vi "Configure Auth.vi"(8 "error in (no error)":errorcluster, 11 "SOL-Server in":refnum<class "SOL-Server.lvclass">) -> (0 "error out":errorcluster, 3 "SOL-Server out":refnum<class "SOL-Server.lvclass">)   [LabVIEW 2020, in "Summer of LabVIEW.lvlib" / "SOL-Server.lvclass"]
uses:
  SOL-Server.lvclass
  <vilib>/IlluminatedG/IG HTTP Server/HTTP Server/Optional Providers.ctl
  <vilib>/IlluminatedG/IG HTTP Server/HTTP Server/Password Encoder/Password Encoder.lvclass
  <vilib>/IlluminatedG/IG HTTP Server/HTTP Server/Authentication Provider/Authentication Provider.lvclass
  SOL-Server.lvclass/SOL-Server.ctl
  <vilib>/IlluminatedG/IG HTTP Server/HTTP Server/FormAuthentication/FormAuthentication.lvclass
  C:/Program Files (x86)/National Instruments/LabVIEW 2020/vi.lib/IlluminatedG/IG HTTP Server/HTTP Server/Authentication Provider/Authentication Provider.lvclass
  User DB/User DB.lvclass
  C:/Program Files (x86)/National Instruments/LabVIEW 2020/vi.lib/IlluminatedG/IG HTTP Server/HTTP Server/User Provider/User Provider.lvclass
  <vilib>/IlluminatedG/IG HTTP Server/HTTP Server/Server/Server.lvclass
  <vilib>/IlluminatedG/IG HTTP Server/HTTP Server/HTTP Server.lvlib
  SOL Auth/SOL Auth.lvclass
  C:/Program Files (x86)/National Instruments/LabVIEW 2020/vi.lib/IlluminatedG/IG HTTP Server/HTTP Server/Service/Service.lvclass
  C:/dev/IlluminatedG/lv-sol-22/SOL Auth/SOL Auth.lvclass
  C:/dev/IlluminatedG/lv-sol-22/User DB/User DB.lvclass
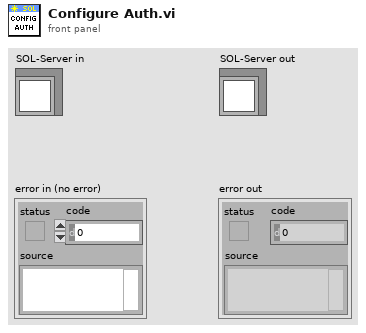
[diagram p1: front panel]
types:
  T1 = typedef "HTTP Server.lvlib/Optional Providers.ctl" = cluster{"Password Encoder":refnum<class "Password Encoder.lvclass">, "Auth":refnum<class "Authentication Provider.lvclass">}
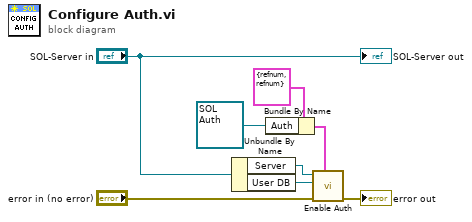
[diagram p0: block diagram]
diagram:
  n1 = Unbundle By Name("SOL-Server in") -> ("Server"=w2:refnum<class "Server.lvclass">, "User DB"=w8:refnum<class "User DB.lvclass">)
  n2 = Bundle By Name(cluster=T1 {"Password Encoder"=refnum, "Auth"=refnum} ("Optional Providers (Basic)"), "Auth"=refnum<class "SOL Auth.lvclass"> refnum ("SOL:SOL Auth.lvclass")) -> (w5:T1)
  n3 = call <vilib>:"Enable Auth.vi"("Optional Providers (Basic)"=w5, "error in (no error)"="error in (no error)", "User Provider"=w8, "Server in"=w2) -> ("error out"=→"error out":errorcluster)  [unwired: 6 in, 1 out]
  "SOL-Server out" <- "SOL-Server in"
